vi "Gif.ApplicationExtension.vi"(0 "data":string, 9 "offset":i32, 11 "error in (no error)":errorcluster) -> (4 "data out":string, 6 "Application Identifier":string, 8 "Application Authentication Code":string, 10 "offset out":i32, 15 "error out":errorcluster)   [LabVIEW 2019]
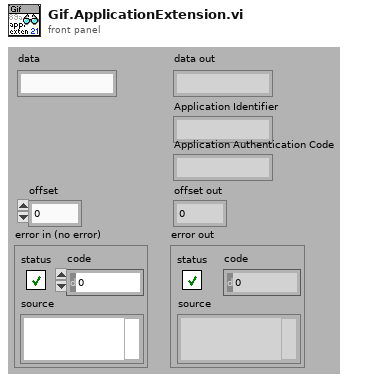
[diagram p1: front panel]
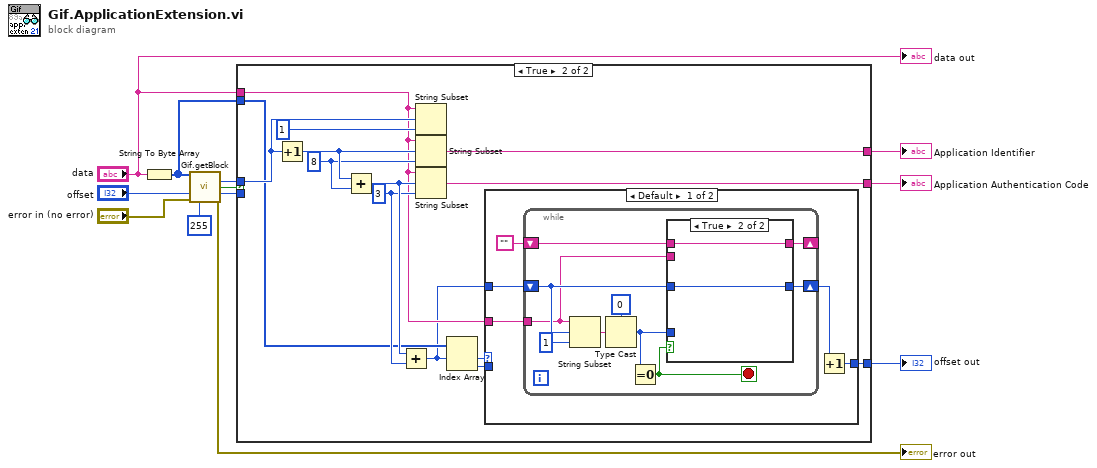
[diagram p0: block diagram]
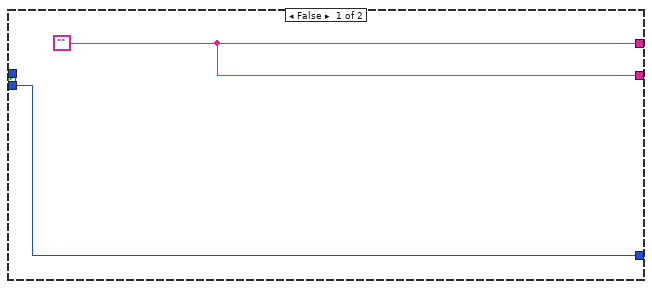
[diagram p2: hidden frame]
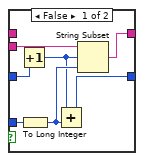
[diagram p3: hidden frame]
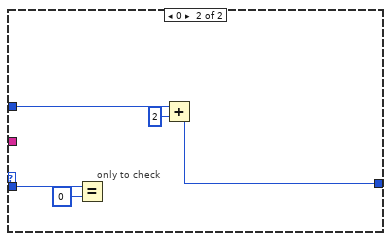
[diagram p4: hidden frame]
diagram:
  n1 = String To Byte Array(string="data") -> (unsigned byte array=w8:u8[])
  n2 = call "Gif.getBlock.vi"("data"=w8, "offset"="offset", "error in (no error)"="error in (no error)", "label"=u8 255 ("element")) -> ("pos offset"=w10:i32, "found?"=w11:bool, "offset out"=w7:i32, "error out"=→"error out":errorcluster)  [unwired: 8 out]
  n3 = case shown="True" w11 {
    tunnel: w10 -> [_ w27]
    tunnel: "data" -> [_ w18]
    tunnel: [w13 w24] -> w9
    tunnel: w8 -> [_ w20]
    tunnel: w7 -> [w14 _]
    tunnel: [w14 w15] -> w6
    tunnel: [w13 w21] -> w5
    frame False {
      w13 = ""
    }
    frame True {
      w22 = 3 ("length (rest)")
      w25 = 8 ("length (rest)")
      n4 = Increment(x=w27) -> (x+1=w26:i32)
      n5 = Add(x=w26, y=w25) -> (x+y=w23:i32)
      n6 = Add(x=w23, y=w22) -> (x+y=w17:i32)
      n7 = String Subset(string=w18, offset (0)=w27, length (rest)=1 ("length (rest)")) -> ()  [unwired: 1 out]
      n8 = String Subset(string=w18, offset (0)=w26, length (rest)=w25) -> (substring=w24:string)
      n9 = String Subset(string=w18, offset (0)=w23, length (rest)=w22) -> (substring=w21:string)
      n10 = Index Array(array=w20, index #1=w17) -> (element #1=w19:u8, element #2=w16:u8)  [unwired: 1 in]
      n11 = case shown="Default" w19 {
        tunnel: w18 -> [w33 _]
        tunnel: w17 -> [w32 w55]
        tunnel: w16 -> [_ w57]
        tunnel: [w30 w53] -> w15
        frame Default {
          n12 = while {
            tunnel: w33 -> [w36]
            shift-right: [w37] -> w31
            shift-left: w32 -> [w38]
            shift-right: [w35] -> _
            shift-left: "" -> [w34]
            stop <- w40 stop-if-true
            n13 = String Subset(string=w36, offset (0)=w38, length (rest)=1 ("length (rest)")) -> (substring=w42:string)
            n14 = Type Cast(type=u8 0 ("element"), x=w42) -> (*(type *) &x=w39:u8)
            n15 = Equal To 0?(x=w39) -> (x = 0?=w40:bool)
            n16 = case shown="True" w40 {
              tunnel: w39 -> [w50 _]
              tunnel: w38 -> [w47 w52]
              tunnel: [w49 w52] -> w37
              tunnel: w36 -> [w48 _]
              tunnel: [w44 w51] -> w35
              tunnel: w34 -> [_ w51]
              frame False {
                n17 = Increment(x=w47) -> (x+1=w45:i32)
                n18 = To Long Integer(number=w50) -> (32bit integer=w46:i32)
                n19 = Add(x=w45, y=w46) -> (x+y=w49:i32)
                n20 = String Subset(string=w48, offset (0)=w45, length (rest)=w46) -> (substring=w44:string)
              }
              frame True {
              }
            }
          }
          n21 = Increment(x=w31) -> (x+1=w30:i32)
        }
        frame 0 {
          # "only to check"
          n22 = Equal?(x=w57, y=u8 0 ("element")) -> ()  [unwired: 1 out]
          n23 = Add(x=w55, y=2) -> (x+y=w53:i32)
        }
      }
    }
  }
  "Application Identifier" <- w9
  "offset out" <- w6
  "Application Authentication Code" <- w5
  "data out" <- "data"
